vi "runscenario run Query.vi"(6 "User Information":T1, 8 "error in (no error)":errorcluster, 10 "sxScenarioId (\"\")":string, 11 "Connection Refnum In":T3) -> (0 "error out":errorcluster, 1 "template keys":T2, 3 "Connection Refnum Out":T3)   [LabVIEW 2011]
uses:
  SI.LIB/ODBC/SQL Controls/Connection Refnum.ctl
  Addons/internet/utils/keyedarr.llb/Keyed Array.ctl
  server/database/Users/User Record.ctl
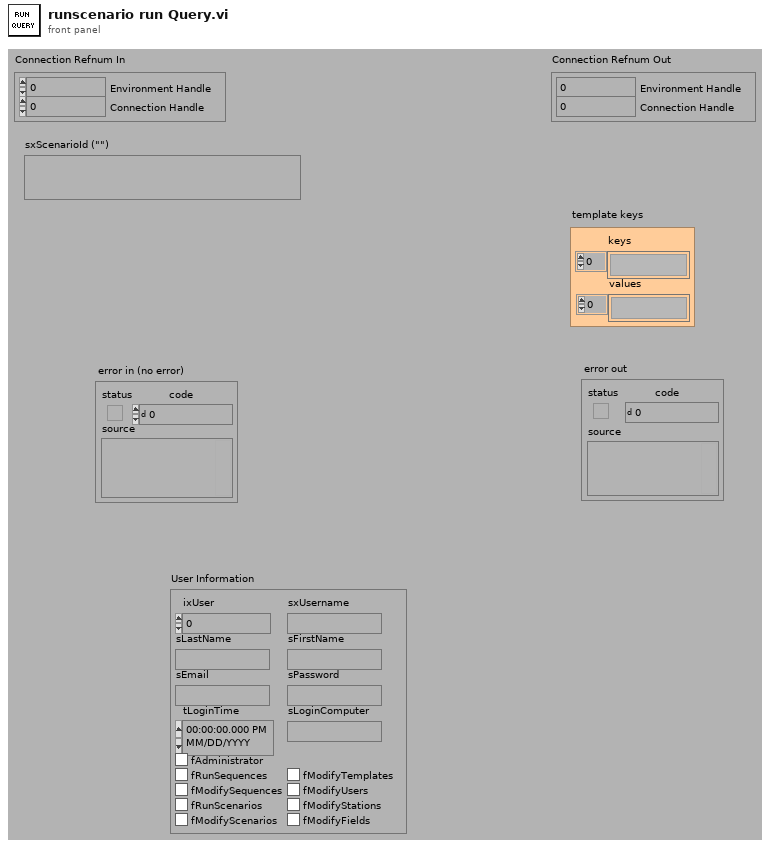
[diagram p1: front panel]
types:
  T1 = typedef "User Record.ctl" = cluster{"ixUser":i32, "sxUsername":string, "sLastName":string, "sFirstName":string, "sEmail":string, "sPassword":string, "tLoginTime":timestamp, "sLoginComputer":string, "fAdministrator":bool, "fRunSequences":bool, "fModifySequences":bool, "fRunScenarios":bool, "fModifyScenarios":bool, "fModifyTemplates":bool, "fModifyUsers":bool, "fModifyStations":bool, "fModifyFields":bool}
  T2 = typedef "Keyed Array.ctl" = cluster{"keys":string[], "values":string[]}
  T3 = typedef "Connection Refnum.ctl" = cluster{"Environment Handle":i32, "Connection Handle":i32}
  T4 = typedef "Scenario Record.ctl" = cluster{"ixScenario":i32, "tCreated":timestamp, "tModified":timestamp, "sxUsername":string, "sModifiedBy":string, "sxScenarioId":string, "sDescription":string, "sLogic":string, "sResultFieldsCSV":string, "sTemplatesCSV":string, "fAutoRunReports":bool, "fSortByTemplates":bool, "fCombinePDF":bool, "Conditions":T5[]}
  T5 = typedef "Condition Record.ctl" = cluster{"iConditionIndex":i32, "sxFieldId":string, "nOperator":T6, "sMatchValue":string}
  T6 = typedef "Condition Operators.ctl" = enum16{"equal (=)", "not equal (\\u2260)", "less than (<)", "less than or equal (\\u2264)", "greater than (>)", "greater than or equal (\\u2265)", "contains", "does not contain"}
  T7 = typedef "Template Record.ctl" = cluster{"ixTemplate":i32, "sxTemplateId":string, "sDescription":string, "sCreator":string, "tCreationDate":timestamp, "sModifier":string, "tModifiedDate":timestamp, "sType":string, "sStyle":string, "sFormat":string, "dWidth":dbl, "dHeight":dbl, "sFilename":string, "sScript":string, "sLayout":string, "sEditor":string, "sStyleProcess":string}
  T8 = typedef "Field Record.ctl" = cluster{"ixField":i32, "iSequenceOrder":i32, "sxFieldId":string, "sxSequenceId":string, "sDisplayName":string, "sValue":string, "sUnits":string, "nDataType":T9, "nNextItem":T10, "fSystem":bool, "fSystemValue":bool, "fRequired":bool, "fSetAtTest":bool, "fTestField":bool, "fDeleted":bool, "fIndexed":bool, "fFreeList":bool}
  T9 = typedef "Field DataTypes.ctl" = enum32{"text", "numeric", "list", "timestamp", "boolean"}
  T10 = typedef "Field NextItem.ctl" = enum32{"Reset", "Retain", "Auto-Increment"}
  T11 = typedef "TDM_INDEX Record.ctl" = cluster{"Model Number":string, "SN for sort":i32, "Test Type":string, "Test Run":string, "Serial Number":string, "Start Timestamp":timestamp, "Data File":path, "Result Columns":string[]}
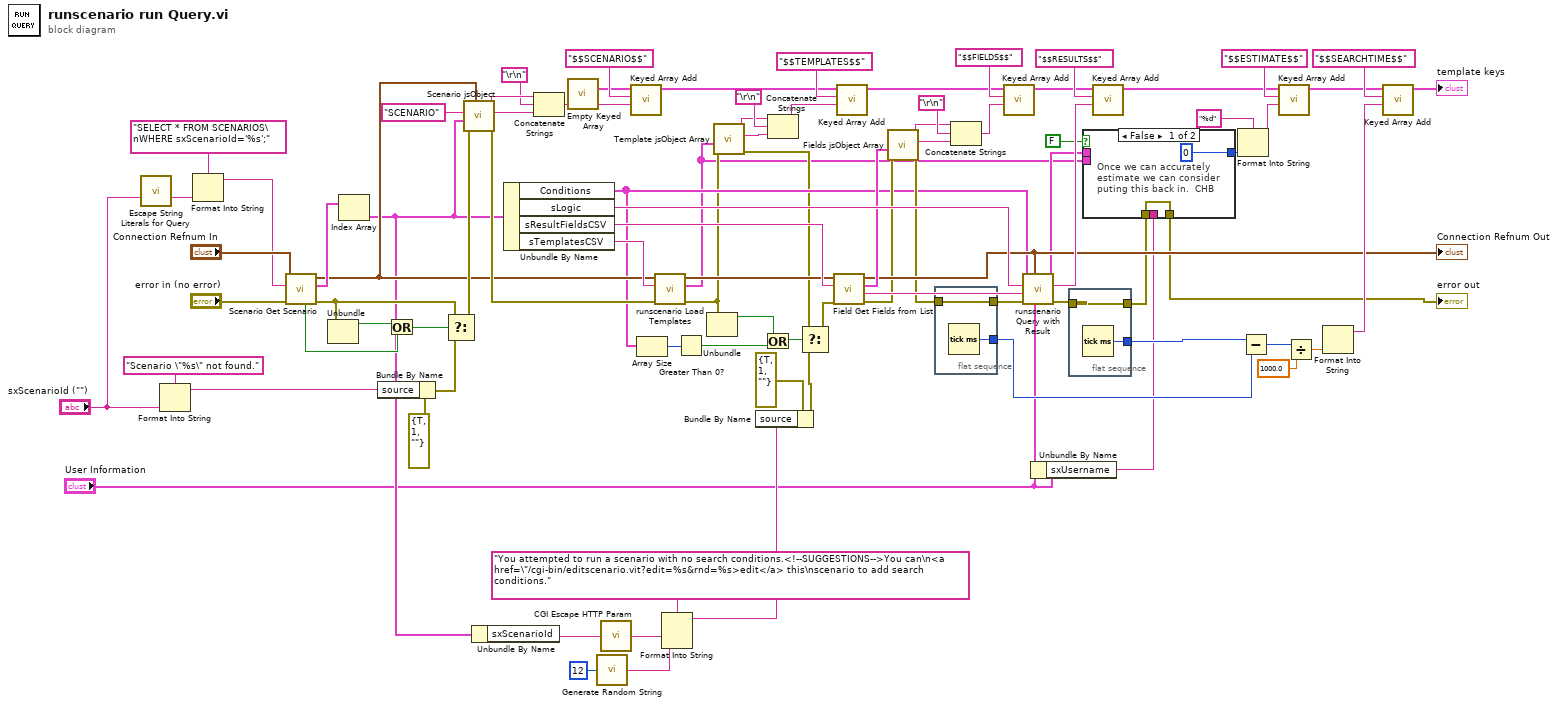
[diagram p0: block diagram]
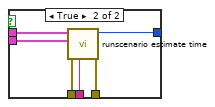
[diagram p2: hidden frame]
diagram:
  n1 = call "Escape String Literals for Query.vi"("String"="sxScenarioId (\"\")") -> ("escaped String"=w77:string)  [unwired: 1 in, 13 out]
  n2 = Format Into String(format string="Scenario \"%s\" not found.", "sxScenarioId (\"\")") -> (resulting string=w86:string)  [unwired: 2 in, 1 out]
  n3 = Format Into String(format string="SELECT * FROM SCENARIOS\nWHERE sxScenarioId='%s';", w77) -> (resulting string=w75:string)  [unwired: 2 in, 1 out]
  n4 = call "Scenario Get Scenario.vi"("error in (no error)"="error in (no error)", "Query"=w75, "Connection Refnum"="Connection Refnum In") -> ("error out"=w81:errorcluster, "Scenarios"=w89:T4[], "Connection Refnum"=w28:T3, "Data Present?"=w79:bool)  [unwired: 5 out]
  n5 = Unbundle(w81) -> ("status"=w80:bool)  [unwired: 2 out]
  n6 = Index Array(array=w89) -> (element=w13:T4)  [unwired: 1 in]
  n7 = Bundle By Name(cluster=errorcluster {"status"=TRUE, "code"=1, "source"=""} ("f"), "source"=w86) -> (w87:errorcluster)
  n8 = Or(x=w80, y=w79) -> (x .or. y?=w78:bool)
  n9 = Select(t=w81, s=w78, f=w87) -> (s? t:f=w52:errorcluster)
  n10 = call "Scenario jsObject.vi"("Connection Refnum"=w28, "error in (no error)"=w52, "Scenario Record (empty)"=w13, "Scenario jsObject Name (\"\")"="SCENARIO" ("Scenario jsObject Name (\"\")")) -> ("error out"=w51:errorcluster, "Scenario jsObject"=w48:string, "SCENARIO jsObject Definition"=w50:string)  [unwired: 2 in, 3 out]
  n11 = Unbundle By Name(w13) -> ("sxScenarioId"=w12:string)
  n12 = Unbundle By Name(w13) -> ("Conditions"=w26:T5[], "sLogic"=w71:string, "sResultFieldsCSV"=w63:string, "sTemplatesCSV"=w58:string)
  n13 = Concatenate Strings(w50, "\r\n", w48) -> (w47:string)
  n14 = call "Empty Keyed Array.vi"() -> ("empty keyed array"=w53:T2)  [unwired: 3 out]
  n15 = call "Generate Random String.vi"("String Length (5)"=12) -> ("Output String"=w15:string)  [unwired: 4 out]
  n16 = call "CGI Escape HTTP Param.vi"("string"=w12) -> ("url-encoded string"=w14:string)
  n17 = call "Keyed Array Add.vi"("value"=w47, "key"="$$SCENARIO$$", "array in"=w53) -> ("array out"=w36:T2)  [unwired: 1 in, 3 out]
  n18 = Array Size(array=w26) -> (size(s)=w27:i32)
  n19 = call "runscenario Load Templates.vi"("error in (no error)"=w51, "TemplateCSV (\"\")"=w58, "Connection Refnum"=w28) -> ("error out"=w21:errorcluster, "Templates"=w8:T7[], "Connection Refnum"=w59:T3)  [unwired: 1 in, 5 out]
  n20 = Format Into String(format string="You attempted to run a scenario with no search conditions.<!--SUGGESTIONS-->You can\n<a href=\"/cgi-bin/editscenario.vit?edit=%s&rnd=%s>edit</a> this\nscenario to add search conditions." ("source"), w14, w15) -> (resulting string=w11:string)  [unwired: 2 in, 1 out]
  n21 = Greater Than 0?(x=w27) -> (x > 0?=w18:bool)
  n22 = Unbundle(w21) -> ("status"=w19:bool)  [unwired: 2 out]
  n23 = call "Template jsObject Array.vi"("error in (no error)"=w21, "TEMPLATES (none)"=w8) -> ("error out"=w25:errorcluster, "Templates jsObject Array"=w33:string, "Template jsObject Definition"=w32:string)  [unwired: 2 in, 5 out]
  n24 = Bundle By Name(cluster=errorcluster {"status"=TRUE, "code"=1, "source"=""} ("f"), "source"=w11) -> (w23:errorcluster)
  n25 = Or(x=w19, y=w18) -> (x .or. y?=w20:bool)
  n26 = Concatenate Strings(w32, "\r\n", w33) -> (w31:string)
  n27 = Select(t=w25, s=w20, f=w23) -> (s? t:f=w24:errorcluster)
  n28 = call "Field Get Fields from List.vi"("error in (no error)"=w24, "sxFieldIdsCSV (\"\")"=w63, "Connection Refnum"=w59) -> ("error out"=w30:errorcluster, "new Fields CSV"=w60:string, "Fields"=w61:T8[], "Connection Refnum"=w56:T3)  [unwired: 5 out]
  "Connection Refnum Out" <- w56
  n29 = call "Keyed Array Add.vi"("value"=w31, "key"="$$TEMPLATES$$", "array in"=w36) -> ("array out"=w35:T2)  [unwired: 1 in, 3 out]
  n30 = call "Fields jsObject Array.vi"("error in (no error)"=w30, "FIELDS (none)"=w61) -> ("error out"=w29:errorcluster, "Fields jsObject Array"=w43:string, "Field jsObject Definition"=w44:string)  [unwired: 2 in, 5 out]
  n31 = flat-sequence {
    tunnel: w29 -> [w91]
    tunnel: [w91] -> w70
    tunnel: [w90] -> w66
    frame #0 {
      n32 = Tick Count (ms)() -> (millisecond timer value=w90:u32)
    }
  }
  n33 = Concatenate Strings(w44, "\r\n", w43) -> (w42:string)
  n34 = call "Keyed Array Add.vi"("value"=w42, "key"="$$FIELDS$$", "array in"=w35) -> ("array out"=w39:T2)  [unwired: 1 in, 3 out]
  n35 = call "runscenario Query with Result.vi"("User"="User Information", "Connection Refnum"=w56, "error in (no error)"=w70, "Result FieldIds CSV (\"\")"=w60, "Logic String (\"\": AND all conditions)"=w71, "Conditions (none)"=w26) -> ("error out"=w4:errorcluster, "jsResults"=w64:string, "runs"=w9:T11[])  [unwired: 3 out]
  n36 = Unbundle By Name("User Information") -> ("sxUsername"=w6:string)
  n37 = flat-sequence {
    tunnel: w4 -> [w93]
    tunnel: [w93] -> w3
    tunnel: [w92] -> w67
    frame #0 {
      n38 = Tick Count (ms)() -> (millisecond timer value=w92:u32)
    }
  }
  n39 = case shown="False" FALSE {
    tunnel: w9 -> [_ w101]
    tunnel: w8 -> [_ w100]
    tunnel: w6 -> [_ w99]
    tunnel: [0 ("estimate (secs)") w98] -> w5
    tunnel: w3 -> [w95 w97]
    tunnel: [w95 w96] -> w2
    frame False {
      # "Once we can accurately\nestimate we can consider\nputing this back in.  CHB"
    }
    frame True {
      n40 = call "runscenario estimate time.vi"("User"=w99, "error in (no error)"=w97, "Templates"=w100, "runs"=w101) -> ("error out"=w96:errorcluster, "estimate (secs)"=w98:i32)  [unwired: 6 out]
    }
  }
  "error out" <- w2
  n41 = call "Keyed Array Add.vi"("value"=w64, "key"="$$RESULTS$$", "array in"=w39) -> ("array out"=w41:T2)  [unwired: 1 in, 3 out]
  n42 = Format Into String(format string="%d", w5) -> (resulting string=w38:string)  [unwired: 2 in, 1 out]
  n43 = Subtract(x=w67, y=w66) -> (x-y=w69:u32)
  n44 = call "Keyed Array Add.vi"("value"=w38, "key"="$$ESTIMATE$$", "array in"=w41) -> ("array out"=w40:T2)  [unwired: 1 in, 3 out]
  n45 = Divide(x=w69, y=1000.0 ("number (0 to 1)")) -> (x/y=w65:dbl)
  n46 = Format Into String(w65) -> (resulting string=w72:string)  [unwired: 3 in, 1 out]
  n47 = call "Keyed Array Add.vi"("value"=w72, "key"="$$SEARCHTIME$$", "array in"=w40) -> ("array out"=→"template keys":T2)  [unwired: 1 in, 3 out]
